vi "Erase Curve.vi"(8 "error in (no error)":errorcluster, 10 "Curve to Erase (21)":dbl=21.0, 11 "VISA resource name":refnum<visa-resource-name>) -> (0 "error out":errorcluster, 3 "VISA resource name out":refnum<visa-resource-name>)   [LabVIEW 2019, in "Lake Shore 325.lvlib"]
doc: "This VI erases a user curve. Erasing the curve sets all identification parameters to default and blanks all breakpoint values."
uses:
  Lake Shore 325.lvlib
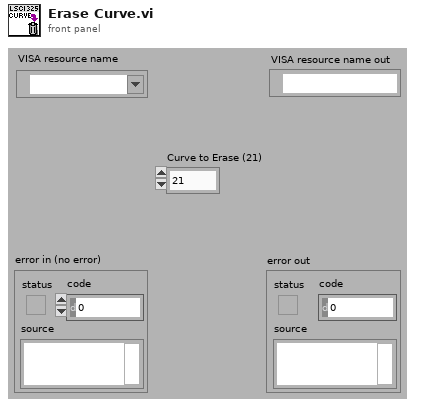
[diagram p1: front panel]
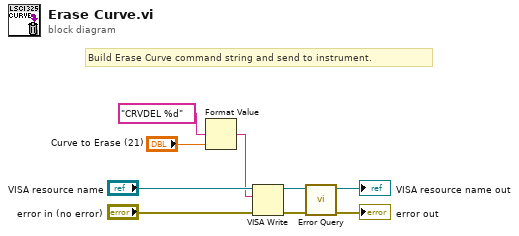
[diagram p0: block diagram]
diagram:
  # "Build Erase Curve command string and send to instrument."
  n1 = Format Value(format string="CRVDEL %d", value (0)="Curve to Erase (21)") -> (output string=w2:string)  [unwired: 1 in]
  n2 = VISA Write(VISA resource name="VISA resource name", write buffer=w2, error in (no error)="error in (no error)") -> (VISA resource name out=w6:refnum<visa-resource-name>, error out=w7:errorcluster)  [unwired: 1 out]
  n3 = call "Error Query.vi"("error in (no error)"=w7, "VISA resource name"=w6) -> ("error out"=→"error out":errorcluster, "VISA resource name out"=→"VISA resource name out":refnum<visa-resource-name>)  [unwired: 7 in, 1 out]
